vi "Pre-Init.vi"(8 "error in (no error)":errorcluster, 11 "LR-700 Driver in":refnum<class "LR-700 Driver.lvclass">) -> (0 "error out":errorcluster, 3 "LR-700 Driver out":refnum<class "LR-700 Driver.lvclass">)   [LabVIEW 2015, in "LR-700 Driver.lvclass"]
uses:
  LR-700 Driver.lvclass
  VISA Instrument/VISA Instrument.lvclass
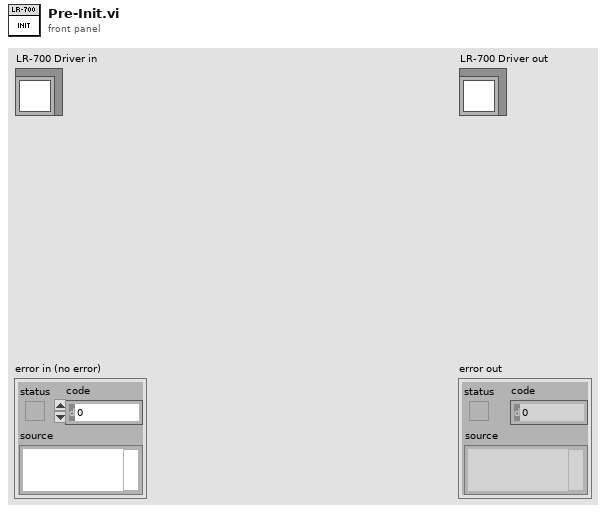
[diagram p1: front panel]
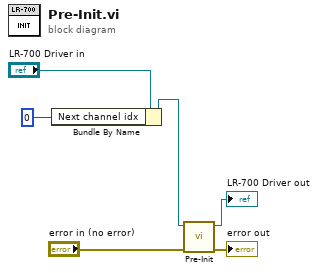
[diagram p0: block diagram]
diagram:
  n1 = Bundle By Name(cluster="LR-700 Driver in", "Next channel idx"=0) -> (w2:refnum<class "LR-700 Driver.lvclass">)
  n2 = call-parent "Pre-Init.vi"("error in (no error)"="error in (no error)", "Instrument Driver in"=w2) -> ("error out"=→"error out":errorcluster, "Instrument Driver out"=→"LR-700 Driver out":refnum<class "LR-700 Driver.lvclass">)  [unwired: 8 in]
